vi "Write to DB.vi"(8 "error in (no error)":errorcluster, 11 "Database Entry in":refnum<class "Database Entry.lvclass">) -> (0 "error out":errorcluster, 3 "Database Entry out":refnum<class "Database Entry.lvclass">)   [LabVIEW 2021, in "Database Entry.lvclass"]
uses:
  Database Entry.lvclass
  Database Entry.lvclass/Database Entry.ctl
  <vilib>/Utility/file.llb/Read Delimited Spreadsheet (string).vi
  <vilib>/Utility/file.llb/Write Delimited Spreadsheet (string).vi
  Components/Stack/Stack.lvclass
panel:
  out "Final name":string
  out "Data cluster":T1={"module or proto"="proto", " geometry"="full", "resolution"="LD", "baselayer"="BA_123", "toplayer"="SI_789", "bl_pos"="1", "tl_pos"="1", "put_pos"="1", "region"="1", "asstray"="1", "comptray"="1", "put"="1", "date"="2024-04-02", "timestart"="1:12:12.442", "timeend"="1:23:45.244", "operator"="cmuperson", "tape"="some", "glue"="some", "stack name"="some"}
  out "error out py":errorcluster
  out "String Out":string="Upload Success"
  in  "error in (no error) py":errorcluster
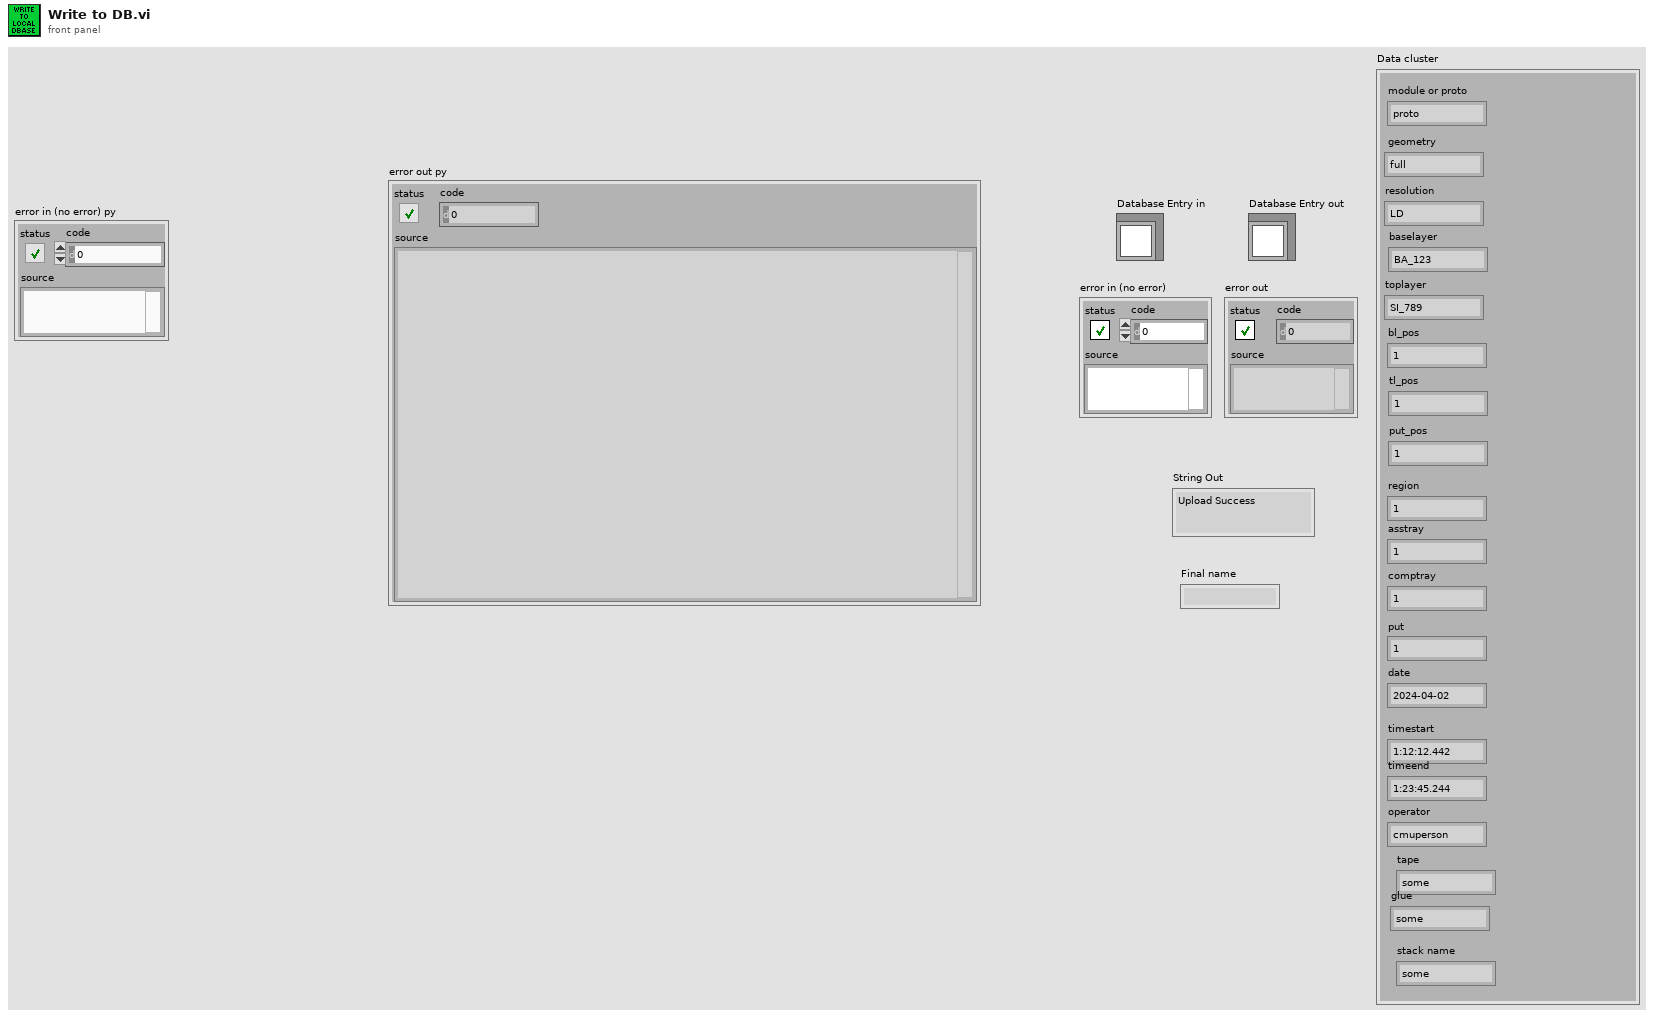
[diagram p1: front panel]
types:
  T1 = cluster{"module or proto":string, " geometry":string, "resolution":string, "baselayer":string, "toplayer":string, "bl_pos":string, "tl_pos":string, "put_pos":string, "region":string, "asstray":string, "comptray":string, "put":string, "date":string, "timestart":string, "timeend":string, "operator":string, "tape":string, "glue":string, "stack name":string}
  T2 = typedef "File Paths.ctl" = cluster{"Glue Pattern Folder":path, "Carrier Tray Folder":path, "Pick Up Tool Fixture Folder":path, "Components Folder":path, "Bellows Tool Offset.txt":path, "Pick Up Tool Offset.txt":path, "Dispense Tip Offset.txt":path, "Log Files":path, "Gantry Assembly Map.txt":path, "Syringe and offset map.txt":path, "Controllers Folder":path, "Local dbase config":path}
  T3 = cluster{"type":string, " geometry":string, "resolution":string, "baselayer":string, "toplayer":string, "bl_pos":string, "tl_pos":string, "put_pos":string, "region":string, "asstray":string, "comptray":string, "put":string, "date":string, "timestart":string, "timeend":string, "operator":string, "tape":string, "glue":string, "stack name":string}
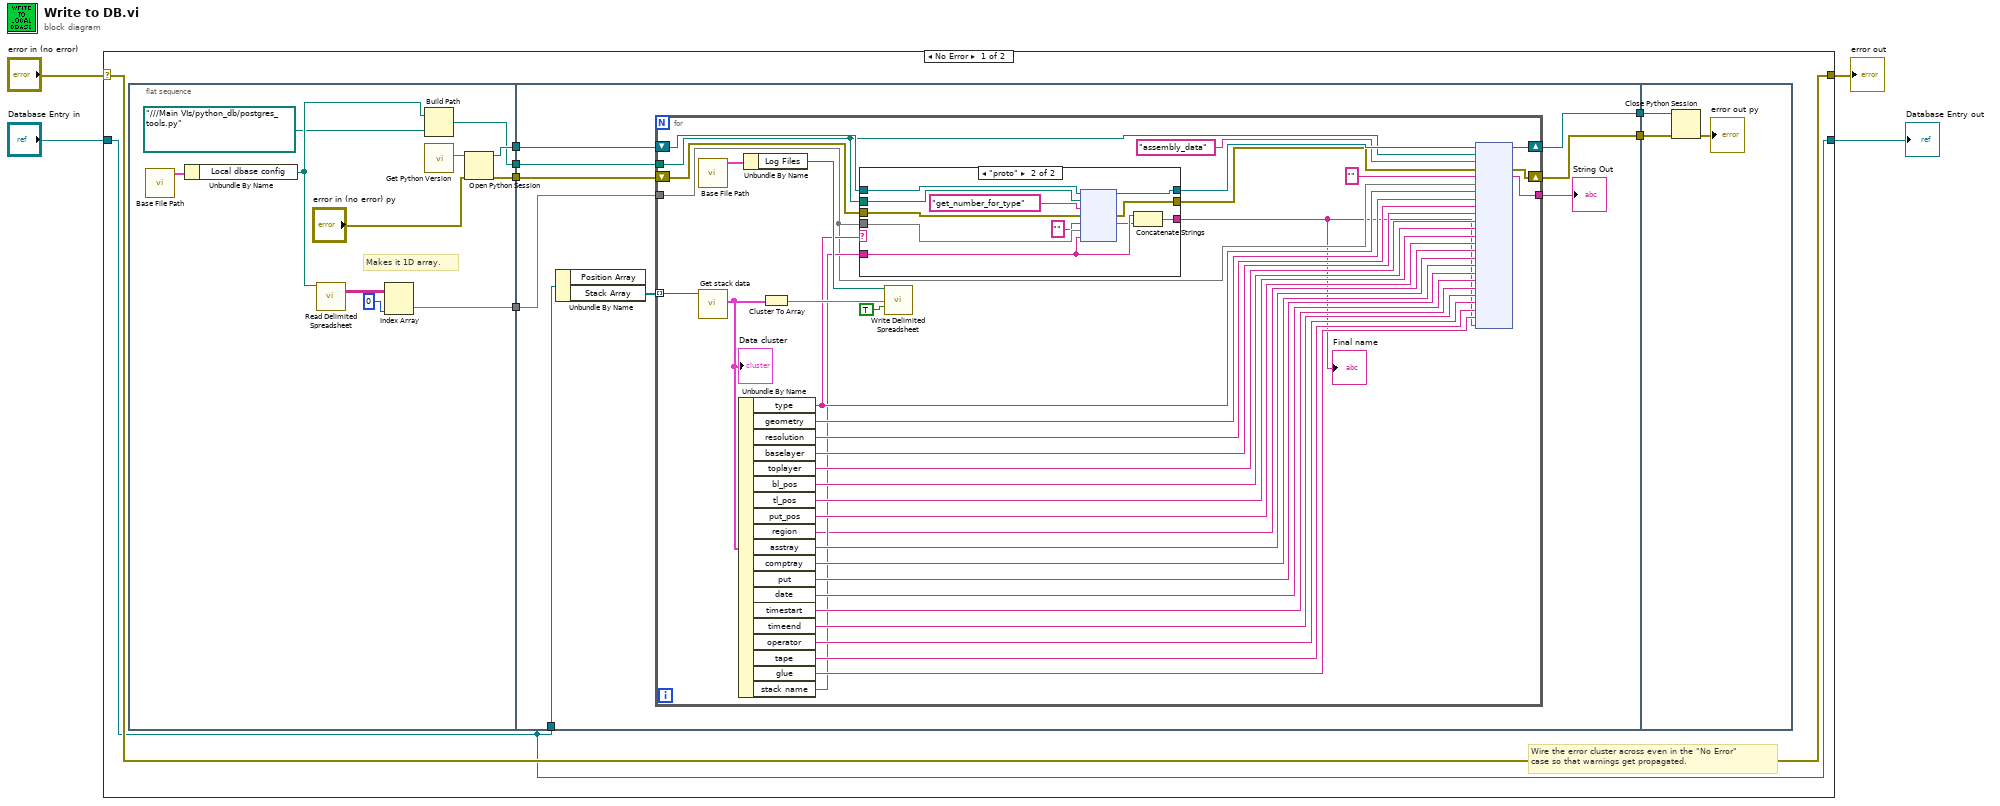
[diagram p0: block diagram]
diagram:
  n1 = case shown="No Error" "error in (no error)" {
    selector: "error in (no error)" -> [w12 w88]
    tunnel: [w12 w88] -> w3
    tunnel: [w5 w87] -> w1
    tunnel: "Database Entry in" -> [w5 w87]
    frame No Error {
      # "Wire the error cluster across even in the \"No Error\"\ncase so that warnings get propagated."
      n2 = flat-sequence {
        tunnel: [w22] -> w11
        tunnel: [w23] -> w10
        tunnel: [w19] -> w9
        tunnel: [w15] -> w8
        tunnel: [w31] -> w7
        tunnel: [w30] -> w6
        tunnel: w11 -> [w32]
        tunnel: w10 -> [w29]
        tunnel: w9 -> [w28]
        tunnel: w8 -> [w27]
        tunnel: w5 -> [w26]
        tunnel: w7 -> [w85]
        tunnel: w6 -> [w86]
        frame #0 {
          # "Makes it 1D array."
          n3 = call "Base File Path.vi"() -> ("Paths Out"=w20:T2)  [unwired: 11 in]
          n4 = Unbundle By Name(w20) -> ("Local dbase config"=w18:path)
          n5 = call-poly <vilib>:"Read Delimited Spreadsheet.vi"("file path (dialog if empty)"=w18) -> ("all rows"=w17:string[][])  [unwired: 9 in, 5 out]
          n6 = Index Array(array=w17, index (col)=0 ("disabled index (col)")) -> (element=w15:string[])  [unwired: 1 in]
          n7 = Build Path(base path=w18, name or relative path=path "../../../Main VIs/python_db/postgres_tools.py" ("module path")) -> (appended path=w19:path)
          n8 = call "Get Python Version.vi"() -> ("Python Version"=w13:string)  [unwired: 10 in, 1 out]
          n9 = Open Python Session(python version=w13, 3:"error in (no error) py") -> (session out=w23:refnum<k35>, error out=w22:errorcluster)  [unwired: 1 in]
        }
        frame #1 {
          n10 = Unbundle By Name(w26) -> ("Stack Array"=w24:refnum<class "Stack.lvclass">[])  [unwired: 1 out]
          n11 = for {
            tunnel: w28 -> [w38]
            shift-right: [w69] -> w31
            shift-left: w32 -> [w37]
            shift-right: [w68] -> w30
            shift-left: w29 -> [w40]
            tunnel: [w67] -> w25
            tunnel: w24 -> [w66] mode=indexing
            tunnel: w27 -> [w41]
            n12 = call "Base File Path.vi"() -> ("Paths Out"=w46:T2)  [unwired: 11 in]
            n13 = call "Get stack data.vi"("Stack in"=w66) -> ("Data cluster"=w44:T3)  [unwired: 8 in, 2 out]
            "Data cluster" <- w44
            n14 = Unbundle By Name(w44) -> ("type"=w43:string, "geometry"=w64:string, "resolution"=w63:string, "baselayer"=w62:string, "toplayer"=w61:string, "bl_pos"=w60:string, "tl_pos"=w59:string, "put_pos"=w58:string, "region"=w34:string, "asstray"=w57:string, "comptray"=w56:string, "put"=w55:string, "date"=w54:string, "timestart"=w53:string, "timeend"=w52:string, "operator"=w51:string, "tape"=w50:string, "glue"=w49:string, "stack name"=w42:string)
            n15 = Unbundle By Name(w46) -> ("Log Files"=w45:path)
            n16 = Cluster To Array(cluster=w44) -> (array=w48:string[])
            n17 = case shown="\"proto\"" w43 {
              tunnel: w42 -> [w72 w81]
              tunnel: [w72 w83] -> w33
              tunnel: w41 -> [_ w82]
              tunnel: w40 -> [w71 w80]
              tunnel: [w71 w79] -> w39
              tunnel: w38 -> [_ w77]
              tunnel: w37 -> [w70 w76]
              tunnel: [w70 w75] -> w36
              frame "module", Default {
              }
              frame "proto" {
                n18 = node(w80, w77, "get_number_for_type" ("function name"), w76, "" ("function name"), w82, w81) -> (w79:refnum<k35>, w75:errorcluster, w73:string)  [unwired: 2 in, 2 out]
                n19 = Concatenate Strings(w81, w73) -> (w83:string)
              }
            }
            "Final name" <- w33
            n20 = call-poly <vilib>:"Write Delimited Spreadsheet.vi"("file path (dialog if empty)"=w45, "1D data"=w48, "append to file? (new file:F)"=TRUE) -> ()  [unwired: 11 in, 2 out]
            n21 = node(w39, w38, "assembly_data" ("function name"), w36, "", w41, w43, w64, w63, w62, w61, w60, w59, w58, w34, w57, w56, w55, w54, w53, w52, w51, w50, w49, w33) -> (w68:refnum<k35>, w69:errorcluster, w67:string)  [unwired: 20 in, 2 out]
          }
          "String Out" <- w25
        }
        frame #2 {
          n22 = Close Python Session(session in=w86, error in=w85) -> (11:→"error out py":errorcluster)
        }
      }
    }
    frame Error {
    }
  }
  "error out" <- w3
  "Database Entry out" <- w1
